vi "Request Data JSON.vi"(8 "error in (no error)":errorcluster, 11 "BatchRequest in":refnum<class "BatchRequest.lvclass">) -> (0 "error out":errorcluster, 2 "Request Data JSON":string, 3 "BatchRequest out":refnum<class "BatchRequest.lvclass">)   [LabVIEW 2022 SP3, in "obs-websocket-lv.lvlib" / "BatchRequest.lvclass"]
uses:
  BatchRequest.lvclass
  BatchRequest.lvclass/BatchRequest.ctl
  Request/Request.lvclass
  <vilib>/IlluminatedG/lv-web-crypto/lv-json/JSON/JSON.lvlib
  C:/dev/illuminatedg/obs-websocket-lv/obs-websocket-lv/Request/Request.lvclass
  C:/dev/illuminatedg/obs-websocket-lv/obs-websocket-lv/Client Message/Client Message.lvclass
  C:/dev/illuminatedg/obs-websocket-lv/obs-websocket-lv/Message/Message.lvclass
  C:/dev/illuminatedg/obs-websocket-lv/obs-websocket-lv/BatchRequest/BatchRequest.lvclass
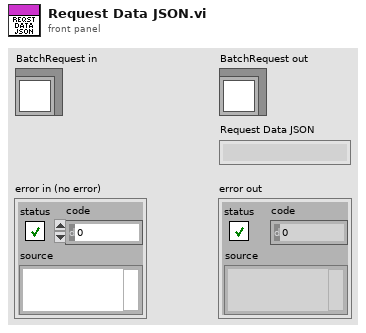
[diagram p1: front panel]
types:
  T1 = typedef "obs-websocket-lv.lvlib/Batch Execution Type.ctl" = i16
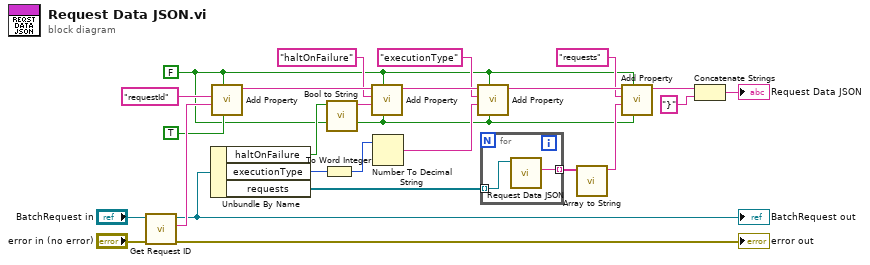
[diagram p0: block diagram]
diagram:
  w1 = FALSE ("Include Empty?")
  n1 = call "Get Request ID.vi"("error in (no error)"="error in (no error)", "Request in"="BatchRequest in") -> ("error out"=→"error out":errorcluster, "Request ID"=w22:string, "Request out"=w3:refnum<class "BatchRequest.lvclass">)  [unwired: 7 in]
  "BatchRequest out" <- w3
  n2 = Unbundle By Name(w3) -> ("haltOnFailure"=w20:bool, "executionType"=w18:T1, "requests"=w11:refnum<class "Request.lvclass">[])
  n3 = call <vilib>:"Add Property.vi"("String?"=TRUE, "Include Empty?"=w1, "Value"=w22, "Property Name"="requestId") -> ("String out"=w21:string)  [unwired: 7 in]
  n4 = To Word Integer(number=w18) -> (16bit integer=w17:T1)
  n5 = call <vilib>:"Bool to String.vi"("Boolean"=w20) -> ("Value"=w16:string)  [unwired: 10 in]
  n6 = call <vilib>:"Add Property.vi"("String?"=w1, "Include Empty?"=w1, "Value"=w16, "Property Name"="haltOnFailure", "String In"=w21) -> ("String out"=w14:string)  [unwired: 6 in]
  n7 = Number To Decimal String(number=w17) -> (decimal integer string=w13:string)  [unwired: 1 in]
  n8 = call <vilib>:"Add Property.vi"("String?"=w1, "Include Empty?"=w1, "Value"=w13, "Property Name"="executionType", "String In"=w14) -> ("String out"=w8:string)  [unwired: 6 in]
  n9 = for {
    tunnel: w11 -> [w27] mode=indexing
    tunnel: [w26] -> w10 mode=indexing
    n10 = call-dynamic "Request Data JSON.vi"("Request in"=w27) -> ("Request Data JSON"=w26:string)  [unwired: 8 in, 2 out]
  }
  n11 = call <vilib>:"Array to String.vi"("JSON Strings"=w10) -> ("JSON Array String"=w9:string)  [unwired: 10 in]
  n12 = call <vilib>:"Add Property.vi"("String?"=w1, "Include Empty?"=w1, "Value"=w9, "Property Name"="requests", "String In"=w8) -> ("String out"=w6:string)  [unwired: 6 in]
  n13 = Concatenate Strings(w6, "}" ("string")) -> (→"Request Data JSON":string)
